vi "Load_Cals.vi"() -> ()   [LabVIEW 2020]
uses:
  <vilib>/Rock Robotics/Network Tables/NT Write Boolean.vi
  <vilib>/Utility/xml.llb/Write to XML File(string).vi
  <vilib>/Rock Robotics/Network Tables/NT Write Number.vi
panel:
  in  "Subsystem XML File":path[](array[path])=[path "Cals/Turret.XML", path "Cals/Intake.XML", path "Cals/Magazine.XML", path "Cals/Flywheel.XML", path "Cals/Drive.XML"]
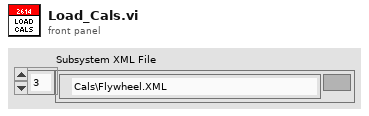
[diagram p1: front panel]
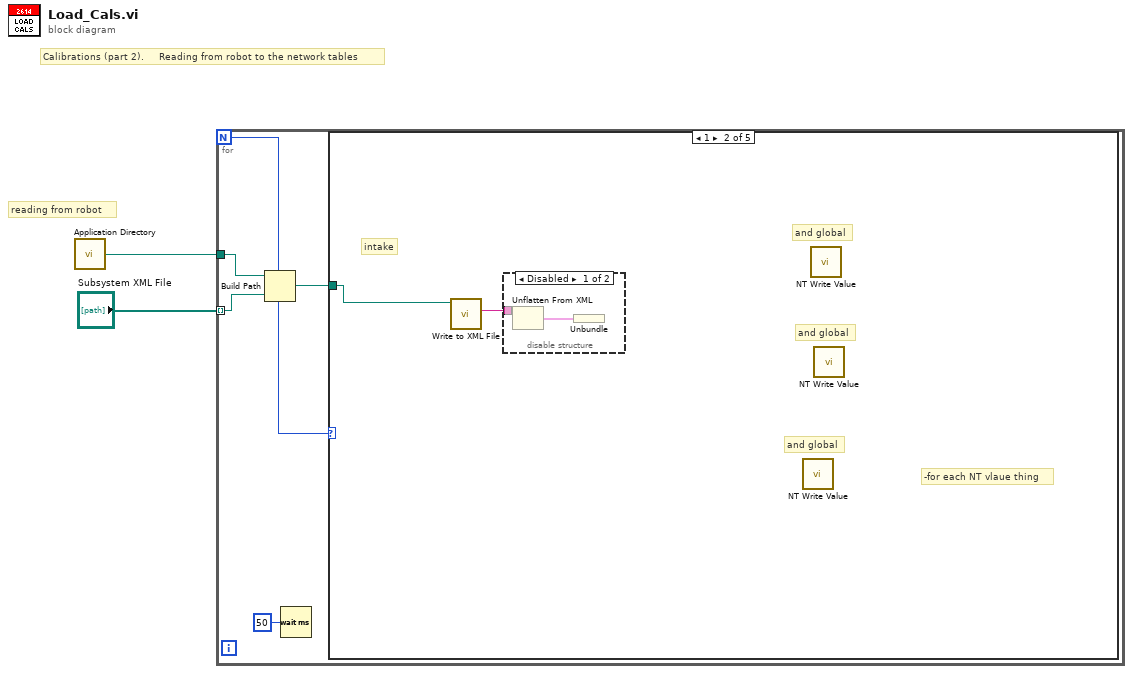
[diagram p0: block diagram]
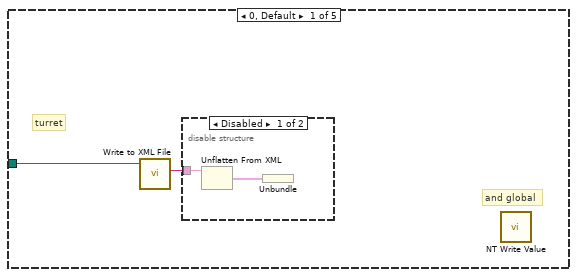
[diagram p2: hidden frame]
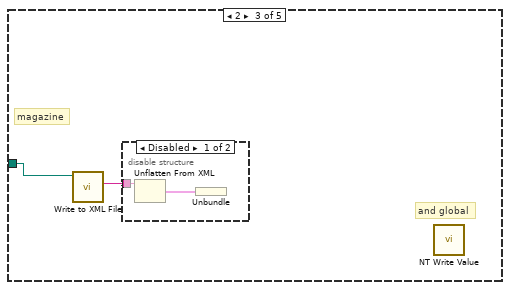
[diagram p5: hidden frame]
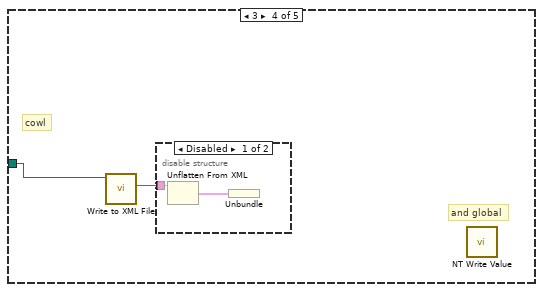
[diagram p7: hidden frame]
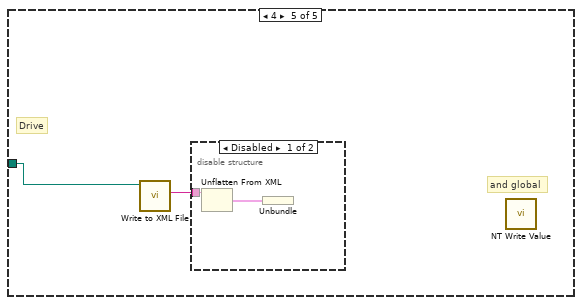
[diagram p9: hidden frame]
diagram:
  # "reading from robot"
  # "Calibrations (part 2).     Reading from robot to the network tables"
  n1 = call <vilib>:"Application Directory.vi"() -> ("Application Directory"=w1:path)
  n2 = for {
    N -> [w7]
    tunnel: "Subsystem XML File" -> [w4] mode=indexing
    tunnel: w1 -> [w3]
    n3 = Build Path(base path=w3, name or relative path=w4) -> (appended path=w5:path)
    n4 = Wait (ms)(milliseconds to wait=u32 50) -> ()  [unwired: 1 out]
    n5 = case shown="1" w7 {
      tunnel: w5 -> [w8 w12 w16 w20 w24]
      frame 0, Default {
        # "and global"
        # "turret"
        n6 = call-poly <vilib>:"Write to XML File.vi"("XML File Path"=w8) -> ("XML String"=w9:string)  [unwired: 8 in, 2 out]
        n7 = disable-structure shown="Disabled" {
          disable-tunnel: w9 -> [w10 _]
          frame Disabled {
            n8 = Unflatten From XML(xml string=w10) -> (value=w11:cluster{})  [unwired: 2 in, 1 out]
            n9 = Unbundle(w11) -> ()  [unwired: 1 out]
          }
          frame Enabled {
          }
        }
        n10 = call-poly <vilib>:"NT Write Value.vi"() -> ()  [unwired: 11 in, 1 out]
      }
      frame 1 {
        # "-for each NT vlaue thing"
        # "and global"
        # "and global"
        # "and global"
        # "intake"
        n11 = call-poly <vilib>:"Write to XML File.vi"("XML File Path"=w12) -> ("XML String"=w13:string)  [unwired: 8 in, 2 out]
        n12 = disable-structure shown="Disabled" {
          disable-tunnel: w13 -> [w14 _]
          frame Disabled {
            n13 = Unflatten From XML(xml string=w14) -> (value=w15:cluster{})  [unwired: 2 in, 1 out]
            n14 = Unbundle(w15) -> ()  [unwired: 1 out]
          }
          frame Enabled {
          }
        }
        n15 = call-poly <vilib>:"NT Write Value.vi"() -> ()  [unwired: 11 in, 1 out]
        n16 = call-poly <vilib>:"NT Write Value.vi"() -> ()  [unwired: 11 in, 1 out]
        n17 = call-poly <vilib>:"NT Write Value.vi"() -> ()  [unwired: 11 in, 1 out]
      }
      frame 2 {
        # "and global"
        # "magazine"
        n18 = call-poly <vilib>:"Write to XML File.vi"("XML File Path"=w16) -> ("XML String"=w17:string)  [unwired: 8 in, 2 out]
        n19 = disable-structure shown="Disabled" {
          disable-tunnel: w17 -> [w18 _]
          frame Disabled {
            n20 = Unflatten From XML(xml string=w18) -> (value=w19:cluster{})  [unwired: 2 in, 1 out]
            n21 = Unbundle(w19) -> ()  [unwired: 1 out]
          }
          frame Enabled {
          }
        }
        n22 = call-poly <vilib>:"NT Write Value.vi"() -> ()  [unwired: 11 in, 1 out]
      }
      frame 3 {
        # "and global"
        # "cowl"
        n23 = call-poly <vilib>:"Write to XML File.vi"("XML File Path"=w20) -> ("XML String"=w21:string)  [unwired: 8 in, 2 out]
        n24 = disable-structure shown="Disabled" {
          disable-tunnel: w21 -> [w22 _]
          frame Disabled {
            n25 = Unflatten From XML(xml string=w22) -> (value=w23:cluster{})  [unwired: 2 in, 1 out]
            n26 = Unbundle(w23) -> ()  [unwired: 1 out]
          }
          frame Enabled {
          }
        }
        n27 = call-poly <vilib>:"NT Write Value.vi"() -> ()  [unwired: 11 in, 1 out]
      }
      frame 4 {
        # "and global"
        # "Drive"
        n28 = call-poly <vilib>:"Write to XML File.vi"("XML File Path"=w24) -> ("XML String"=w25:string)  [unwired: 8 in, 2 out]
        n29 = disable-structure shown="Disabled" {
          disable-tunnel: w25 -> [w26 _]
          frame Disabled {
            n30 = Unflatten From XML(xml string=w26) -> (value=w27:cluster{})  [unwired: 2 in, 1 out]
            n31 = Unbundle(w27) -> ()  [unwired: 1 out]
          }
          frame Enabled {
          }
        }
        n32 = call-poly <vilib>:"NT Write Value.vi"() -> ()  [unwired: 11 in, 1 out]
      }
    }
  }
